vi "Get Right Menu.vi"(8 "error in (no error)":errorcluster, 10 "ATM State":T2, 11 "ATM View Model in":refnum<class "ATM View Model.lvclass">) -> (0 "error out":errorcluster, 2 "Right Menu":T1, 3 "ATM View Model out":refnum<class "ATM View Model.lvclass">)   [LabVIEW 2020, in "ATM View Model.lvclass"]
uses:
  ATM View Model.lvclass
  ATM Controller/State.ctl
  ATM Controller/ATM Controller.lvclass
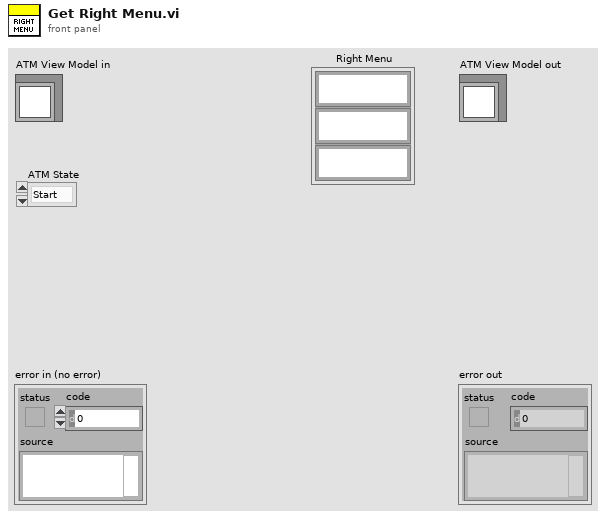
[diagram p1: front panel]
types:
  T1 = cluster{"RFS String":string, "RFS String 2":string, "RFS String 3":string}
  T2 = typedef "ATM Controller.lvclass/State.ctl" = enum16{"Start", "Card Inserted", "Verification Failed", "Verification Succeeded", "Depositing", "Depositing Completed", "Terminate"}
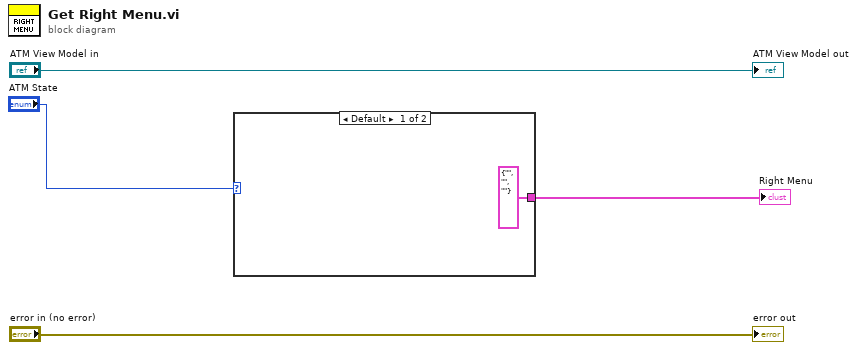
[diagram p0: block diagram]
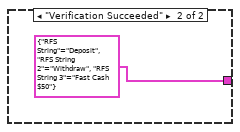
[diagram p2: hidden frame]
diagram:
  n1 = case shown="Default" "ATM State" {
    tunnel: [T1 {"RFS String"="", "RFS String 2"="", "RFS String 3"=""} ("Left Menu") T1 {"RFS String"="Deposit", "RFS String 2"="Withdraw", "RFS String 3"="Fast Cash $50"} ("Left Menu")] -> w1
    frame Default {
    }
    frame "Verification Succeeded" {
    }
  }
  "Right Menu" <- w1
  "error out" <- "error in (no error)"
  "ATM View Model out" <- "ATM View Model in"
